vi "Stop Core.vi"(10 "final error code":i32, 11 "[MDI] Parent in":refnum<class "[MDI] Parent.lvclass">) -> (3 "[MDI] Parent out":refnum<class "[MDI] Parent.lvclass">)   [LabVIEW 2020, in "[MDI] Parent.lvlib" / "[MDI] Parent.lvclass"]
doc: "(<B>Filename</B>: Actor Framework.lvlib:Actor.lvclass:Stop Core.vi)\n\nDefines what the actor does before it stops. Use the <B>final error code</B> input to determine whether the actor shut down in response to an error.\n\nBy default, this method passes the Stop message along to all auto-stop nested actors. A descendant class may override this method to define additional behavior, such as shutting down any processes the actor initiated in its override of the Actor Core method."
uses:
  [MDI] Parent.lvclass
  <vilib>/ActorFramework/Actor/Actor.lvclass
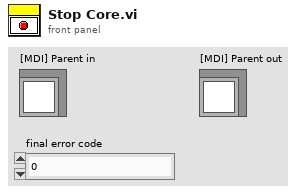
[diagram p1: front panel]
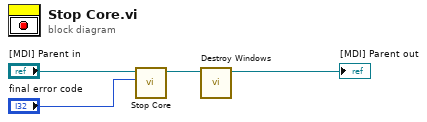
[diagram p0: block diagram]
diagram:
  n1 = call-parent "Stop Core.vi"("final error code"="final error code", "Actor in"="[MDI] Parent in") -> ("Actor out"=w2:refnum<class "[MDI] Parent.lvclass">)  [unwired: 9 in]
  n2 = call "Destroy Windows.vi"("[MDI] Parent in"=w2) -> ("[MDI] Parent out"=→"[MDI] Parent out":refnum<class "[MDI] Parent.lvclass">)  [unwired: 9 in, 1 out]
